vi "list all types.vi"() -> (3 "all types":T1[](array[typedef]))   [LabVIEW 2013, in "data bus tag description.lvclass"]
doc: "A helper function which provides an array of all types supported in the framework."
uses:
  data bus tag description.lvclass
  Data Type.ctl
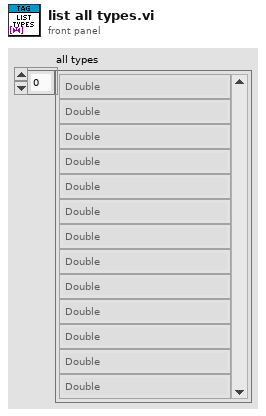
[diagram p1: front panel]
types:
  T1 = typedef "data bus tag description.lvclass/Data Type.ctl" = enum16{"Double", "I64", "Boolean", "Array of Double", "Array of I64", "Variant"}
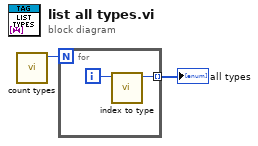
[diagram p0: block diagram]
diagram:
  n1 = call "count types.vi"() -> ("type count"=w1:i32)  [unwired: 11 in]
  n2 = for {
    N: w1 -> [_]
    tunnel: [w4] -> w2 mode=indexing
    i -> [w3]
    n3 = call "index to type.vi"("I32"=w3) -> ("type"=w4:T1)  [unwired: 10 in]
  }
  "all types" <- w2
